vi "Go.vi"(9 "Timing Data":dbl[](array[numeric]), 10 "Control In":T1, 11 "Crosshair Dispense in":refnum<class "Crosshair Dispense.lvclass">) -> (2 "Control Out":T1, 3 "Crosshair Dispense Out":refnum<class "Crosshair Dispense.lvclass">)   [LabVIEW 2019, in "Crosshair Dispense.lvclass"]
uses:
  Crosshair Dispense.lvclass
  Controller/Controllers.ctl
  Controller/I-O/I-O.lvclass
  Controller/Dispenser/Dispenser.lvclass
  C:/Program Files (x86)/Aerotech/A3200/LabVIEW/2010/Bin/Aerotech.A3200.dll
  Program Files (x86)/Aerotech/A3200/LabVIEW/2010/Bin/Aerotech.A3200.dll
  Crosshair Dispense.lvclass/Crosshair Dispense.ctl
  Controller/Motion/A3200/A3200.lvclass
  Controller/Controller.lvclass
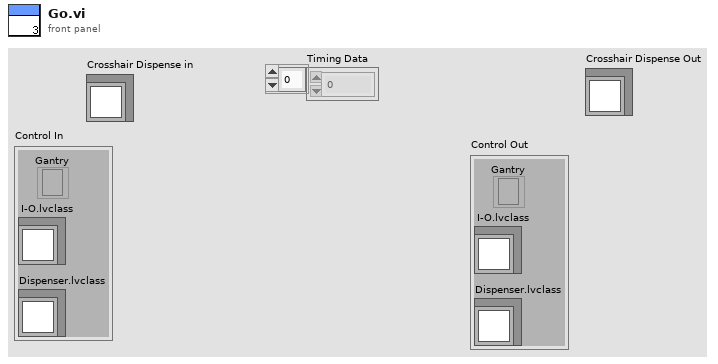
[diagram p1: front panel]
types:
  T1 = typedef "Controller.lvclass/Controllers.ctl" = cluster{"I-O.lvclass":refnum<class "I-O.lvclass">, "Dispenser.lvclass":refnum<class "Dispenser.lvclass">, "Gantry":refnum<k24>}
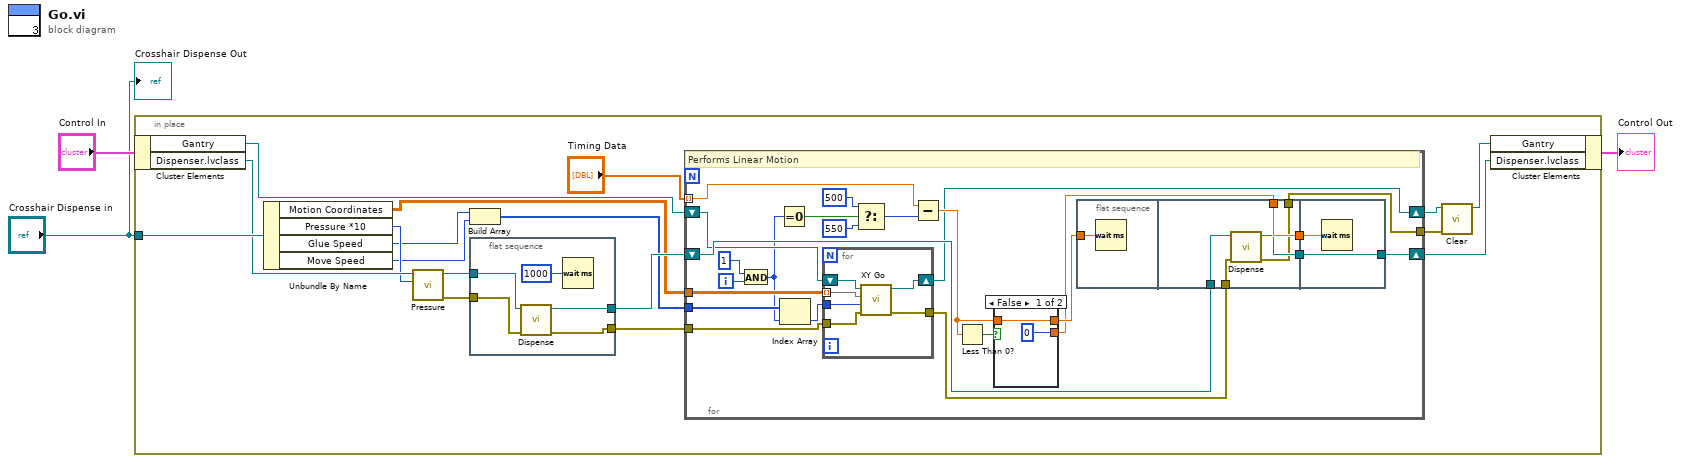
[diagram p0: block diagram]
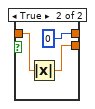
[diagram p2: hidden frame]
diagram:
  n1 = in-place {
    in-place-border: "Crosshair Dispense in" -> [w19]
    n2 = in-place-cluster #1("Control In") -> ("Gantry"=w17:refnum<k24>, "Dispenser.lvclass"=w14:refnum<class "Dispenser.lvclass">)
    n3 = Unbundle By Name(w19) -> ("Motion Coordinates"=w10:dbl[][], "Pressure *10"=w13:i64, "Glue Speed"=w6:i32, "Move Speed"=w5:i32)
    n4 = call-dynamic "Pressure.vi"("Pressure"=w13, "Dispenser in"=w14) -> ("error out"=w12:errorcluster, "Dispenser out"=w11:refnum<class "Dispenser.lvclass">)  [unwired: 8 in]
    n5 = Build Array(w6, w5) -> (w4:i32[])
    n6 = flat-sequence {
      tunnel: [w23] -> w18
      tunnel: w12 -> [w22]
      tunnel: w11 -> [w24]
      tunnel: [w21] -> w9
      frame #0 {
        n7 = call-dynamic "Dispense.vi"("error in (no error)"=w22, "Dispenser in"=w24) -> ("error out"=w21:errorcluster, "Dispenser out"=w23:refnum<class "Dispenser.lvclass">)  [unwired: 8 in]
        n8 = Wait (ms)(milliseconds to wait=u32 1000) -> ()  [unwired: 1 out]
      }
    }
    n9 = for {
      tunnel: w10 -> [w29]
      tunnel: "Timing Data" -> [w41] mode=indexing
      shift-right: [w39] -> w20
      shift-left: w18 -> [w44]
      shift-right: [w38] -> w16
      shift-left: w17 -> [w40]
      tunnel: w9 -> [w32]
      tunnel: [w30] -> w8
      tunnel: w4 -> [w28]
      i -> [w37]
      # "Performs Linear Motion"
      n10 = And(x=1, y=w37) -> (x .and. y?=w27:i32)
      n11 = Equal To 0?(x=w27) -> (x = 0?=w35:bool)
      n12 = Index Array(array=w28, index=w27) -> (element=w26:i32)
      n13 = for {
        shift-right: [w54] -> w38
        shift-left: w40 -> [w55]
        tunnel: w32 -> [w53]
        tunnel: [w52] -> w31
        tunnel: w29 -> [w51] mode=indexing
        tunnel: w26 -> [w50]
        n14 = call "XY Go.vi"("error in (no error)"=w53, "Speed"=w50, "XY"=w51, "Gantry In"=w55) -> ("error out"=w52:errorcluster, "Gantry Out"=w54:refnum<k24>)  [unwired: 6 in]
      }
      n15 = Select(t=500, s=w35, f=550) -> (s? t:f=w43:i32)
      n16 = Subtract(x=w41, y=w43) -> (x-y=w42:dbl)
      n17 = Less Than 0?(x=w42) -> (x < 0?=w49:bool)
      n18 = case shown="False" w49 {
        tunnel: [w65 u32 0 ("milliseconds to wait")] -> w48
        tunnel: w42 -> [w65 w68]
        tunnel: [u32 0 ("milliseconds to wait") w67] -> w47
        frame False {
        }
        frame True {
          n19 = Absolute Value(x=w68) -> (abs(x)=w67:dbl)
        }
      }
      n20 = flat-sequence {
        tunnel: w48 -> [w56]
        tunnel: w44 -> [w60]
        tunnel: [w61] -> w46
        tunnel: w47 -> [w61]
        tunnel: [w59] -> w45
        tunnel: w31 -> [w58]
        tunnel: [w57] -> w30
        tunnel: w46 -> [w63]
        tunnel: w45 -> [w62]
        tunnel: [w62] -> w39
        frame #0 {
          n21 = Wait (ms)(milliseconds to wait=w56) -> ()  [unwired: 1 out]
        }
        frame #1 {
          n22 = call-dynamic "Dispense.vi"("error in (no error)"=w58, "Dispenser in"=w60) -> ("error out"=w57:errorcluster, "Dispenser out"=w59:refnum<class "Dispenser.lvclass">)  [unwired: 8 in]
        }
        frame #2 {
          n23 = Wait (ms)(milliseconds to wait=w63) -> ()  [unwired: 1 out]
        }
      }
    }
    n24 = call "Clear.vi"("error in (no error)"=w8, "Gantry In"=w16) -> ("Gantry Out"=w15:refnum<k24>)  [unwired: 8 in, 1 out]
    n25 = in-place-cluster #1("Gantry"=w15, "Dispenser.lvclass"=w20) -> (→"Control Out":T1)
  }
  "Crosshair Dispense Out" <- "Crosshair Dispense in"
